vi "GetBitfiledValue(Bool).vi"(8 "error in":errorcluster, 10 "bitfield caps":T1={"offset"=0, "size"=0, "signed?"=TRUE}, 11 "register value":u64=9199446298756579247 format="%.0x") -> (0 "error out":errorcluster, 3 "bitfield balue":bool)   [LabVIEW 2015, in "Bitfield.lvlib"]
uses:
  Bitfield.lvlib
  BitfieldCaps.ctl
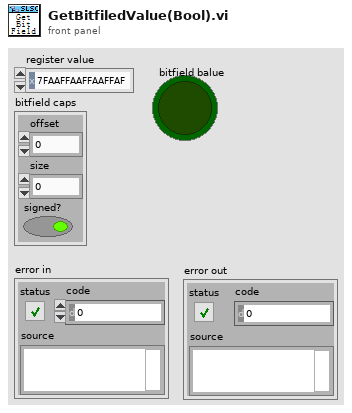
[diagram p1: front panel]
types:
  T1 = typedef "Bitfield.lvlib/BitfieldCaps.ctl" = cluster{"offset":i32, "size":i32, "signed?":bool}
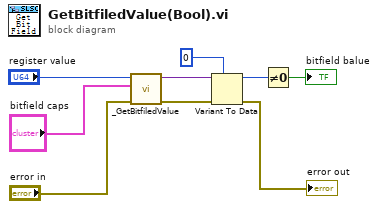
[diagram p0: block diagram]
diagram:
  n1 = call "_GetBitfiledValue.vi"("error in"="error in", "bitfield caps"="bitfield caps", "register value"="register value") -> ("error out"=w5:errorcluster, "bitfield balue"=w8:variant)  [unwired: 7 in]
  n2 = Variant To Data(error in=w5, type=i64 0 ("bitfield balue"), Variant=w8) -> (data=w2:i64, error out=→"error out":errorcluster)
  n3 = Not Equal To 0?(x=w2) -> (x != 0?=→"bitfield balue":bool)
